vi "List Grouped Tags by Type.vi"(8 "error in (no error)":errorcluster, 11 "Group":string) -> (0 "error out":errorcluster, 1 "Tags Out":T1[](array[typedef]))   [LabVIEW 2010, in "Current Value Table.lvlib"]
doc: "This VI will read an entire group as defined during tag creation or by the FormGroup VI. This VI functions as both the normal and static versions of the group read, as the small performance drop from the group name check is insignificant for reasonably sized groups."
uses:
  Current Value Table.lvlib
  Type Defs/Typed Name Set.ctl
  Type Defs/Data Types.ctl
  FGVs/Group Memory Methods.ctl
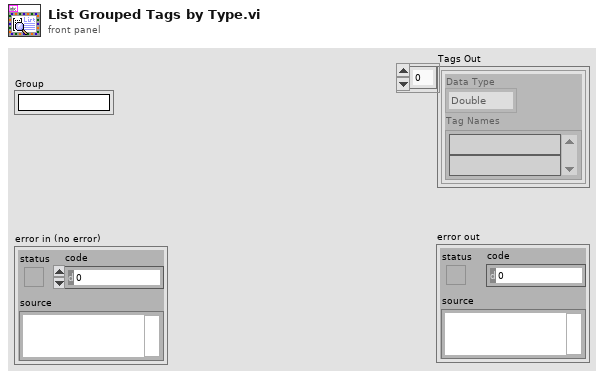
[diagram p1: front panel]
types:
  T1 = typedef "Current Value Table.lvlib/Typed Name Set.ctl" = cluster{"Data Type":T2, "Tag Names":string[]}
  T2 = typedef "Current Value Table.lvlib/Data Types.ctl" = enum16{"Double", "Single", "I64", "I32", "I16", "I8", "U64", "U32", "U16", "U8", "String", "Boolean", "Array of U8", "Array of U16", "Array of U32", "Array of U64", "Array of I64", "Array of I32", "Array of I16", "Array of I8", "Array of Double", "Array of Single", "Array of Boolean", "Array of String"}
  T3 = typedef "Current Value Table.lvlib/Group Memory Methods.ctl" = enum16{"Clear", "Read Indices in Group", "List Groups", "List Tags by Type", "List Tags", "Delete Group", "Check Group Existence", "Create Group"}
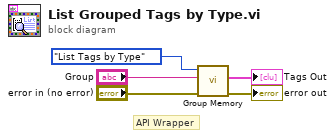
[diagram p0: block diagram]
diagram:
  # "API Wrapper"
  n1 = call "Group Memory.vi"("error in (no error)"="error in (no error)", "Group"="Group", "Method"=Group_Memory_Methods."List Tags by Type") -> ("error out"=→"error out":errorcluster, "Tag Sets Out"=→"Tags Out":T1[])  [unwired: 5 in, 2 out]
